vi "Tag Names.vi"(11 "State In":T1={"State"=enum."Idle", "Start Time"=timestamp(0 s since 1904-01-01), "Configuration"={"Cycle Period"=0.0, "Manual Entry"=0.0, "Output Device"=enum."Default", "EPOS4 Settings"={"VISA resource name"="", "axis"={"keyHandle"=1, "nodeId"=1}, "Simulated?"=FALSE}}, "Current Time"=timestamp(0 s since 1904-01-01), "First Iteration"=FALSE, "Data"={"Centrifuge Speed"=0.0}, "Process Name"="", "Centrifuge On?"=enum."Off", "Output Error"=FALSE, "Log Started"=FALSE}) -> (3 "Centrifuge Module Tag Names":T6, 4 "All Boolean Tags":string[](array[string]), 5 "All  Numeric Tags":string[](array[string]))   [LabVIEW 2018, in "Centrifuge Module.lvlib" / "Centrifuge Module Engine.lvlib"]
uses:
  Centrifuge Module Engine.lvlib
  Centrifuge Module Tag Names Cluster.ctl
  State Cluster.ctl
  State Enum.ctl
  Centrifuge Module Settings Cluster.ctl
  EPOS4/Controls/Device Selection.ctl
  EPOS4/Controls/EPOS Communication Settings.ctl
  Centrifuge Module.lvlib
  EPOS4/EPOS4.lvlib
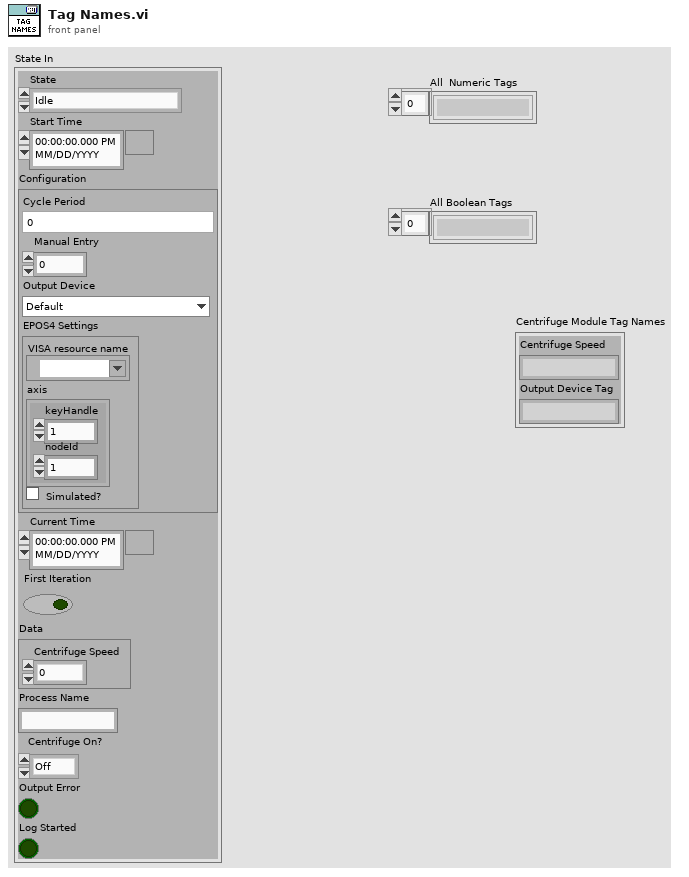
[diagram p1: front panel]
types:
  T1 = typedef "Centrifuge Module.lvlib/Centrifuge Module Engine.lvlib/State Cluster.ctl" = cluster{"State":T2, "Start Time":timestamp, "Configuration":T3, "Current Time":timestamp, "First Iteration":bool, "Data":cluster{"Centrifuge Speed":dbl}, "Process Name":string, "Centrifuge On?":enum16{"Off", "On", "Not Initialized"}, "Output Error":bool, "Log Started":bool}
  T2 = typedef "Centrifuge Module.lvlib/Centrifuge Module Engine.lvlib/State Enum.ctl" = enum16{"Measuring", "Idle", "Paused"}
  T3 = typedef "Centrifuge Module.lvlib/Centrifuge Module Settings Cluster.ctl" = cluster{"Cycle Period":dbl, "Manual Entry":dbl, "Output Device":T4, "EPOS4 Settings":T5}
  T4 = typedef "Device Selection.ctl" = enum16{"Default", "EPOS4"}
  T5 = typedef "EPOS4.lvlib/EPOS Communication Settings.ctl" = cluster{"VISA resource name":refnum<visa-resource-name>, "axis":cluster{"keyHandle":u32, "nodeId":u16}, "Simulated?":bool}
  T6 = typedef "Centrifuge Module.lvlib/Centrifuge Module Tag Names Cluster.ctl" = cluster{"Centrifuge Speed":string, "Output Device Tag":string}
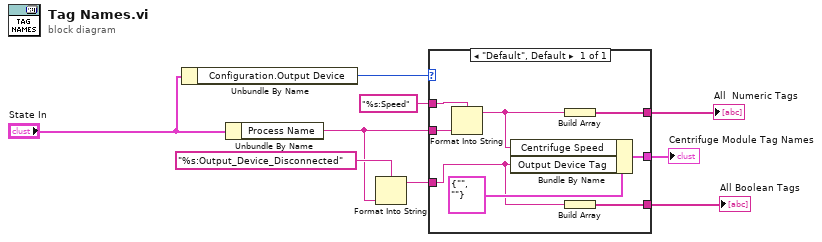
[diagram p0: block diagram]
diagram:
  n1 = Unbundle By Name("State In") -> ("Configuration.Output Device"=w8:T4)
  n2 = Unbundle By Name("State In") -> ("Process Name"=w4:string)
  n3 = Format Into String(format string="%s:Output_Device_Disconnected", w4) -> (resulting string=w2:string)  [unwired: 2 in, 1 out]
  n4 = case shown="\"Default\", Default" w8 {
    tunnel: w4 -> [w16]
    tunnel: w2 -> [w12]
    tunnel: [w17] -> w6
    tunnel: [w14] -> w7
    tunnel: [w11] -> w3
    tunnel: "%s:Speed" ("format string") -> [w10]
    frame "Default", Default {
      n5 = Format Into String(format string=w10, w16) -> (resulting string=w15:string)  [unwired: 2 in, 1 out]
      n6 = Bundle By Name(cluster=T6 {"Centrifuge Speed"="", "Output Device Tag"=""} ("Feed Module Tag Names"), "Centrifuge Speed"=w15, "Output Device Tag"=w12) -> (w14:T6)
      n7 = Build Array(w15) -> (w17:string[])
      n8 = Build Array(w12) -> (w11:string[])
    }
  }
  "Centrifuge Module Tag Names" <- w7
  "All Boolean Tags" <- w3
  "All  Numeric Tags" <- w6
